vi "check.vi"() -> ()   [LabVIEW 2011]
uses:
  <vilib>/express/express arith-compare/Formula/XNode/ExpressFormulaBlockNode.xnode
panel:
  out "arctan(x)":u8
  out "x/y 2":dbl
  out "x/y":dbl
  in  "x 4":u8
  in  "x 3":u8
  in  "x 2":u8
  in  "x":u8
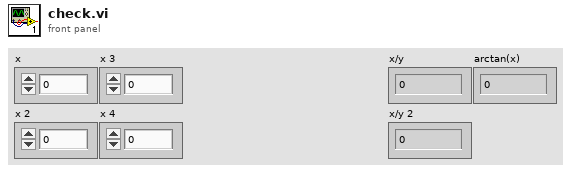
[diagram p1: front panel]
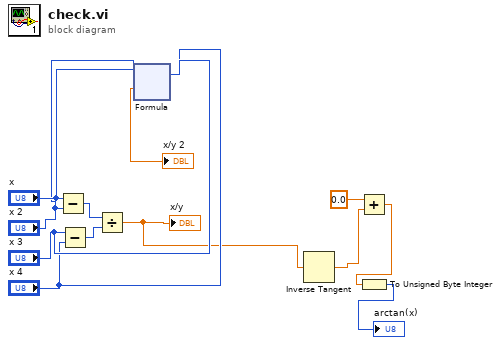
[diagram p0: block diagram]
diagram:
  n1 = Subtract(x="x", y="x 2") -> (x-y=w12:u8)
  n2 = Subtract(x="x 3", y="x 4") -> (x-y=w11:u8)
  n3 = Divide(x=w12, y=w11) -> (x/y=w5:dbl)
  "x/y" <- w5
  n4 = xnode "Formula"("A1"="x", "A2"="x 2", "A3"="x 3", "A4"="x 4") -> ("Result"=→"x/y 2":dbl)  [unwired: 1 in, 1 out]
  n5 = Inverse Tangent(1:w5) -> (0:w3:dbl)
  n6 = Add(x=0.0, y=w3) -> (x+y=w2:dbl)
  n7 = To Unsigned Byte Integer(number=w2) -> (unsigned 8bit integer=→"arctan(x)":u8)
